vi "Logging Settings.vi"(8 "error in (no error)":errorcluster, 11 "Configuration in":refnum<class "Configuration.lvclass">) -> (0 "error out":errorcluster, 3 "Configuration out":refnum<class "Configuration.lvclass">)   [LabVIEW 2017, in "Measurement Actor.lvlib" / "Step Configuration.lvclass"]
uses:
  Step Configuration.lvclass
  <userlib>/Configuration Dialog Actor/Configuration.lvclass
  C:/Program Files (x86)/National Instruments/LabVIEW 2017/user.lib/Configuration Dialog Actor/Configuration.lvclass
  Step Configuration.lvclass/Step Configuration.ctl
  Logger/config/Logger Configuration.lvclass/Logger Configuration.ctl
  Logger/config/Logger Configuration.lvclass
panel:
  in  "Cluster":T1
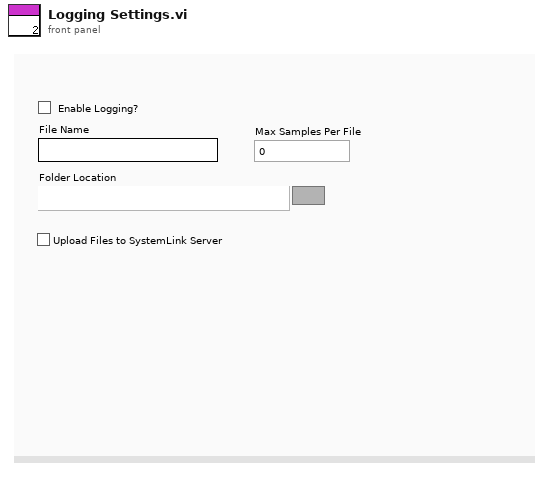
[diagram p1: front panel]
types:
  T1 = cluster{"File Name":string, "Upload Files to SystemLink Server":bool, "Max Samples Per File":dbl, "Folder Location":path, "Logging":bool}
  T2 = cluster{"File Name":string, "Upload Files to SystemLink Server":bool, "Max Samples Per File":i32, "Folder Location":path, "Logging":bool}
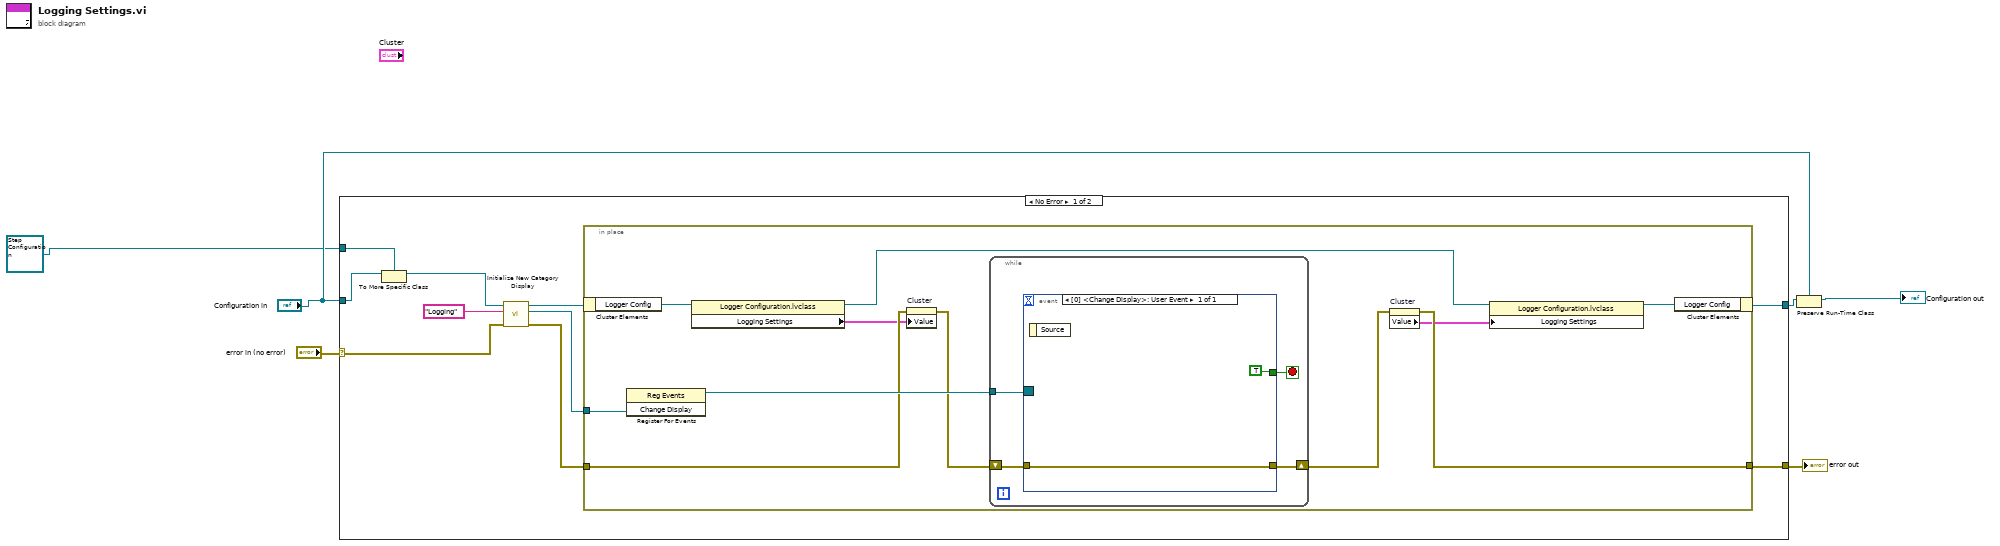
[diagram p0: block diagram]
diagram:
  n1 = case shown="No Error" "error in (no error)" {
    selector: "error in (no error)" -> [w13 w35]
    tunnel: [w12 w34] -> w3
    tunnel: [w7 w35] -> w6
    tunnel: "Configuration in" -> [w10 w34]
    tunnel: refnum<class "Step Configuration.lvclass"> refnum ("Measurement Actor.lvlib:Step Configuration.lvclass") -> [w8 _]
    frame No Error {
      n2 = To More Specific Class(target class=w8, reference=w10) -> (specific class reference=w9:refnum<class "Step Configuration.lvclass">)  [unwired: 1 in, 1 out]
      n3 = call <userlib>:"Initialize New Category Display.vi"("error in (no error)"=w13, "Name to Display"="Logging", "Configuration in"=w9) -> ("error out"=w15:errorcluster, "Change Display"=w16:refnum<user-event>, "Configuration Out"=w11:refnum<class "Step Configuration.lvclass">)  [unwired: 6 in]
      n4 = in-place {
        in-place-border: w16 -> [w27]
        in-place-border: w15 -> [w23]
        in-place-border: [w25] -> w7
        n5 = in-place-cluster #1(w11) -> ("Logger Config"=w21:refnum<class "Logger Configuration.lvclass">)
        n6 = register-events(w27) -> (reference out=w26:refnum<event-registration>)  [unwired: 2 in, 1 out]
        n7 = property class="Logger Configuration.lvclass"(reference=w21) -> (reference out=w17:refnum<class "Logger Configuration.lvclass">, "Logging Settings"=w20:T2)  [unwired: 1 in, 1 out]
        n8 = property on="Cluster" class="Clust (strict)"(error in=w23, "Value"=w20) -> (error out=w22:errorcluster)  [unwired: 1 in, 1 out]
        n9 = while {
          tunnel: w26 -> [w30]
          shift-right: [w29] -> w24
          shift-left: w22 -> [w28]
          stop <- w31 stop-if-true
          n10 = event shown="[0] <Change Display>: User Event" {
            selector: w30 -> [_]
            dyn-events: _ -> [_]
            timeout: _ -> [_]
            tunnel: [TRUE] -> w31
            tunnel: [w32] -> w29
            tunnel: w28 -> [w32]
            event User Event {
              n11 = event-data() -> ()  [unwired: 1 in, 1 out]
            }
          }
        }
        n12 = property on="Cluster" class="Clust (strict)"(error in=w24) -> (error out=w25:errorcluster, "Value"=w19:T1)  [unwired: 1 in, 1 out]
        n13 = property class="Logger Configuration.lvclass"(reference=w17, "Logging Settings"=w19) -> (reference out=w18:refnum<class "Logger Configuration.lvclass">)  [unwired: 1 in, 1 out]
        n14 = in-place-cluster #1("Logger Config"=w18) -> (w12:refnum<class "Step Configuration.lvclass">)
      }
    }
    frame Error {
    }
  }
  "error out" <- w6
  n15 = Preserve Run-Time Class(object in=w3, 2:"Configuration in") -> (object out=→"Configuration out":refnum<class "Configuration.lvclass">)  [unwired: 1 in, 1 out]
